vi "Create Hard Link.vi"(7 "Create Folders? (T)":bool=TRUE, 8 "Error In":errorcluster, 9 "Link Destination Path":path, 10 "Existing File Path":path, 11 "Configuration":T1) -> (0 "Error Out":errorcluster, 2 "Created Hardlink Path":path, 3 "Configuration":T1)   [LabVIEW 2011, in "LVH-Build-Tools.lvlib"]
uses:
  LVH-Build-Tools.lvlib
  Type Defs/Configuration.ctl
  Type Defs/Install Configuration.ctl
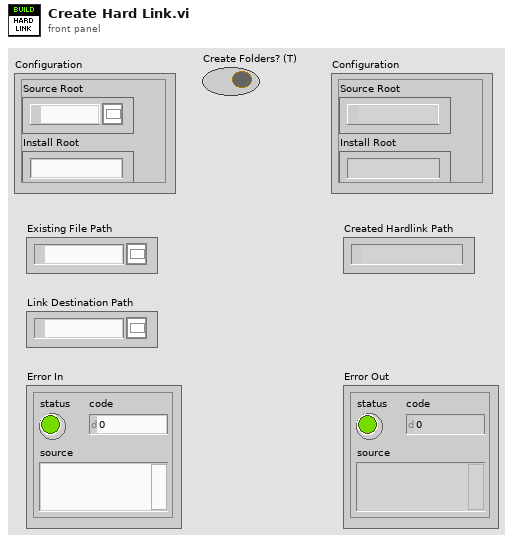
[diagram p1: front panel]
types:
  T1 = typedef "LVH-Build-Tools.lvlib/Configuration.ctl" = cluster{"Source Root":path, "Install Root":string, "Components":string[], "Ignore":string[], "Config Files":path[], "LV Directories":path[], "Install Paths":T2}
  T2 = typedef "LVH-Build-Tools.lvlib/Install Configuration.ctl" = cluster{"LabVIEW Directory":path, "Project Source Config":path}
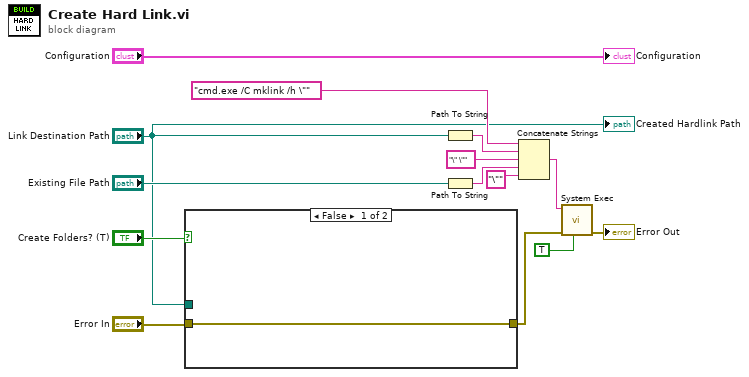
[diagram p0: block diagram]
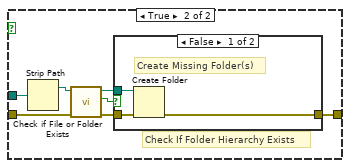
[diagram p2: hidden frame]
diagram:
  n1 = case shown="False" "Create Folders? (T)" {
    tunnel: "Link Destination Path" -> [_ w22]
    tunnel: "Error In" -> [w15 w20]
    tunnel: [w15 w16] -> w2
    frame False {
    }
    frame True {
      # "Check If Folder Hierarchy Exists"
      n2 = Strip Path(path=w22) -> (stripped path=w21:path)  [unwired: 1 out]
      n3 = call <vilib>:"Check if File or Folder Exists.vi"("error in (no error)"=w20, "path"=w21) -> ("error out"=w17:errorcluster, "file or folder exists?"=w19:bool, "dup path"=w18:path)  [unwired: 7 in]
      n4 = case shown="False" w19 {
        tunnel: w18 -> [w25 _]
        tunnel: w17 -> [w24 w26]
        tunnel: [w23 w26] -> w16
        frame False {
          # "Create Missing Folder(s)"
          n5 = Create Folder(path (use dialog)=w25, error in=w24) -> (error out=w23:errorcluster)  [unwired: 1 in, 2 out]
        }
        frame True {
        }
      }
    }
  }
  n6 = Path To String(path="Link Destination Path") -> (string=w8:string)
  n7 = Path To String(path="Existing File Path") -> (string=w10:string)
  n8 = Concatenate Strings("cmd.exe /C mklink /h \"", w8, "\" \"" ("string"), w10, "\"" ("string")) -> (w12:string)
  n9 = call <vilib>:"System Exec.vi"("run minimized? (F)"=TRUE, "error in (no error)"=w2, "command line"=w12) -> ("error out"=→"Error Out":errorcluster)  [unwired: 5 in, 3 out]
  "Configuration" <- "Configuration"
  "Created Hardlink Path" <- "Link Destination Path"
